vi "CASE-ENUM.vi"() -> ()   [LabVIEW 2020]
panel:
  in  "OPCIONES":T1(ring)
  out "Numeric":dbl
  in  "NUMERO  2":dbl
  in  "NUMERO 1":dbl
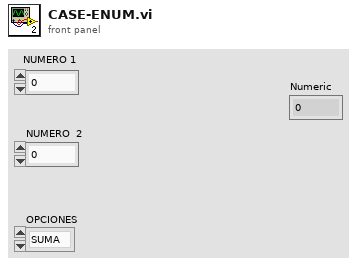
[diagram p1: front panel]
types:
  T1 = enum16{"SUMA", "RESTA", "MULTIPLICACION", "DIVISION"}
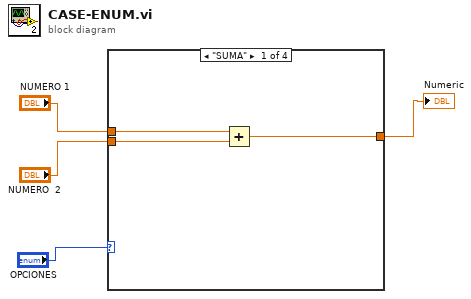
[diagram p0: block diagram]
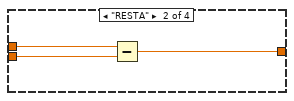
[diagram p2: hidden frame]
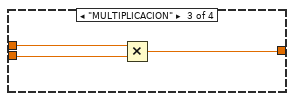
[diagram p3: hidden frame]
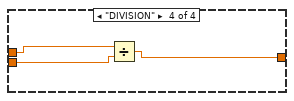
[diagram p4: hidden frame]
diagram:
  n1 = case shown="\"SUMA\"" "OPCIONES" {
    tunnel: [w7 w8 w13 w16] -> w3
    tunnel: "NUMERO 1" -> [w6 w10 w12 w15]
    tunnel: "NUMERO  2" -> [w5 w9 w11 w14]
    frame "SUMA" {
      n2 = Add(x=w6, y=w5) -> (x+y=w7:dbl)
    }
    frame "RESTA" {
      n3 = Subtract(x=w10, y=w9) -> (x-y=w8:dbl)
    }
    frame "MULTIPLICACION" {
      n4 = Multiply(x=w12, y=w11) -> (x*y=w13:dbl)
    }
    frame "DIVISION" {
      n5 = Divide(x=w15, y=w14) -> (x/y=w16:dbl)
    }
  }
  "Numeric" <- w3
